vi "NI VeriStand - Set Custom Device Channel Default Value.vi"(8 "error in (no error)":errorcluster, 10 "Default Value":dbl, 11 "Channel Ref in":T1 format="%.0x") -> (0 "error out":errorcluster, 3 "Channel Ref out":T1=18446744073709551615 format="%.0x")   [LabVIEW 2020, in "Custom Device Offline API.lvlib"]
uses:
  <vilib>/NI VeriStand/Custom Device Offline API/Custom Device Offline API.lvlib
  <vilib>/NI VeriStand/Custom Device API/Custom Device Item Ref.ctl
  NationalInstruments.VeriStand.SystemDefinitionAPI
  <vilib>/NI VeriStand/Custom Device API/Custom Device API.lvlib
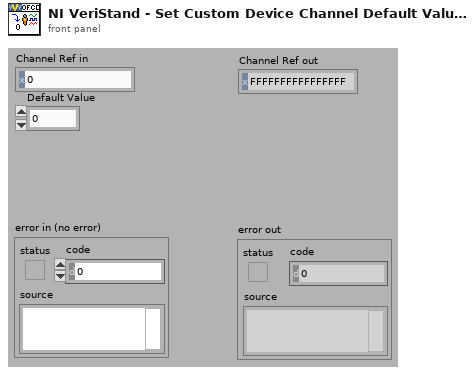
[diagram p1: front panel]
types:
  T1 = typedef "Custom Device API.lvlib/Custom Device Item Ref.ctl" = u64
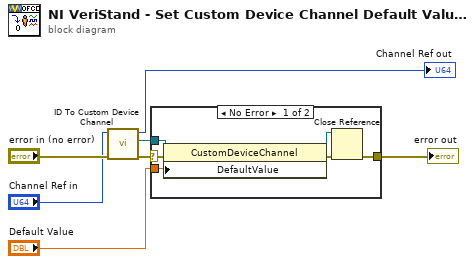
[diagram p0: block diagram]
diagram:
  n1 = call <vilib>:"ID To Custom Device Channel.vi"("error in (no error)"="error in (no error)", "ID in"="Channel Ref in") -> ("error out"=w7:errorcluster, "Channel"=w6:refnum<k24>, "ID out"=→"Channel Ref out":u64)  [unwired: 7 in]
  n2 = case shown="No Error" w7 {
    selector: w7 -> [w11 w14]
    tunnel: w6 -> [w13 _]
    tunnel: "Default Value" -> [w12 _]
    tunnel: [w8 w14] -> w1
    frame No Error {
      n3 = property class="CustomDeviceChannel"(reference=w13, error in=w11, "DefaultValue"=w12) -> (reference out=w9:refnum<k24>, error out=w10:errorcluster)
      n4 = Close Reference(reference=w9, error in (no error)=w10) -> (error out=w8:errorcluster)
    }
    frame Error {
    }
  }
  "error out" <- w1
